vi "Unregister and Close Sessions.vi"(8 "error in":errorcluster) -> (0 "error out":errorcluster)   [LabVIEW 2021, in "NI-Switch Control Relay.lvlib"]
doc: "This VI will get called as part of the TestStand ProcessCleanup sequence. It unregisters and destroys all Switch sessions in the Session Management Service."
uses:
  NI-Switch Control Relay.lvlib
  <vilib>/Plug-In SDKs/Clients/Session Management V1/Session Reservation/Initialize and Close Session Behavior.ctl
  <vilib>/Plug-In SDKs/Clients/Session Management V1/Session Reservation/Session Reservation.lvclass
  Source/Sessions/niSwitch/Session Management niSwitch.lvlib
  <instrlib>/niSwitch/niSwitch.llb/niSwitch Topologies.ctl
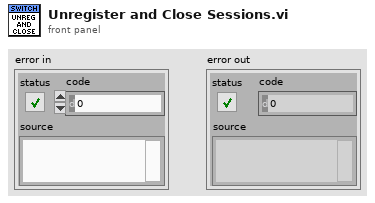
[diagram p1: front panel]
types:
  T1 = typedef "niSwitch Topologies.ctl" = string
  T2 = typedef "NI Session Management V1 Client.lvlib/Session Reservation.lvclass/Initialize and Close Session Behavior.ctl" = enum16{"Auto", "Initialize and Close", "Attach and Detach", "Initialize and Detach", "Attach and Close"}
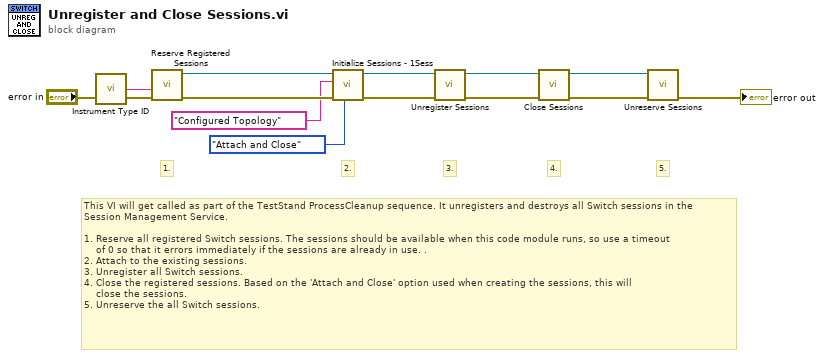
[diagram p0: block diagram]
diagram:
  # "3."
  # "5."
  # "4."
  # "2."
  # "1."
  # "This VI will get called as part of the TestStand ProcessCleanup sequence. It unregisters and destroys all Switch sessions in the\nSession Management Service.\n\n1. Reserve all registered Switch sessions. The sessions should be available when this code module runs, so use a timeout\n    of 0 so that it errors immediately if the sessions are already in use. .\n2. Attach to the existing sessions.\n3. Unregister all Switch sessions.\n4. Close the registered sessions. Based on the 'Attach and Close' option used when creating the sessions, this will\n    close the sessions.\n5. Unreserve the all Switch sessions."
  n1 = call "Instrument Type ID.vi"() -> ("instrument type id"=w5:string)  [unwired: 5 in]
  n2 = call <vilib>:"Reserve Registered Sessions.vi"("error in"="error in", "instrument type id"=w5) -> ("error out"=w3:errorcluster, "session reservation out"=w4:refnum<class "Session Reservation.lvclass">)  [unwired: 8 in]
  n3 = call "Initialize Sessions - 1Sess.vi"("initialize and close session behavior"=Initialize_and_Close_Session_Behavior."Attach and Close", "error in"=w3, "topology name"=T1 "Configured Topology", "session reservation in"=w4) -> ("error out"=w13:errorcluster, "session reservation out"=w9:refnum<class "Session Reservation.lvclass">)  [unwired: 4 in, 2 out]
  n4 = call <vilib>:"Unregister Sessions.vi"("error in"=w13, "session reservation in"=w9) -> ("error out"=w12:errorcluster, "session reservation out"=w8:refnum<class "Session Reservation.lvclass">)  [unwired: 8 in]
  n5 = call <vilib>:"Close Sessions.vi"("error in"=w12, "session reservation in"=w8) -> ("error out"=w11:errorcluster, "session reservation out"=w7:refnum<class "Session Reservation.lvclass">)  [unwired: 8 in]
  n6 = call <vilib>:"Unreserve Sessions.vi"("error in"=w11, "session reservation in"=w7) -> ("error out"=→"error out":errorcluster)  [unwired: 9 in]
